vi "BinanceAPI_roundToPattern.vi"(0 "Value to round":ext, 5 "Value Pattern ( only 0 or 1 - e.g.  0,001 )":dbl) -> (4 "Rounded Value":dbl, 6 "dokladnosc zaokraglenia":i32)   [LabVIEW 2022 SP3]
doc: "Program dodatkowy\n\n\nProgram ten zaokrągla liczbę <B>Value to round</B> do tego miejsca po przecinku co podany przykład czyli <B>Value Pattern</B>"
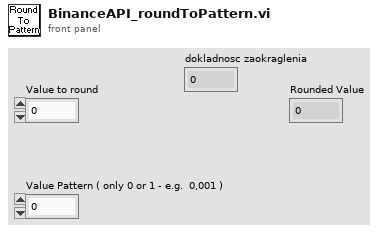
[diagram p1: front panel]
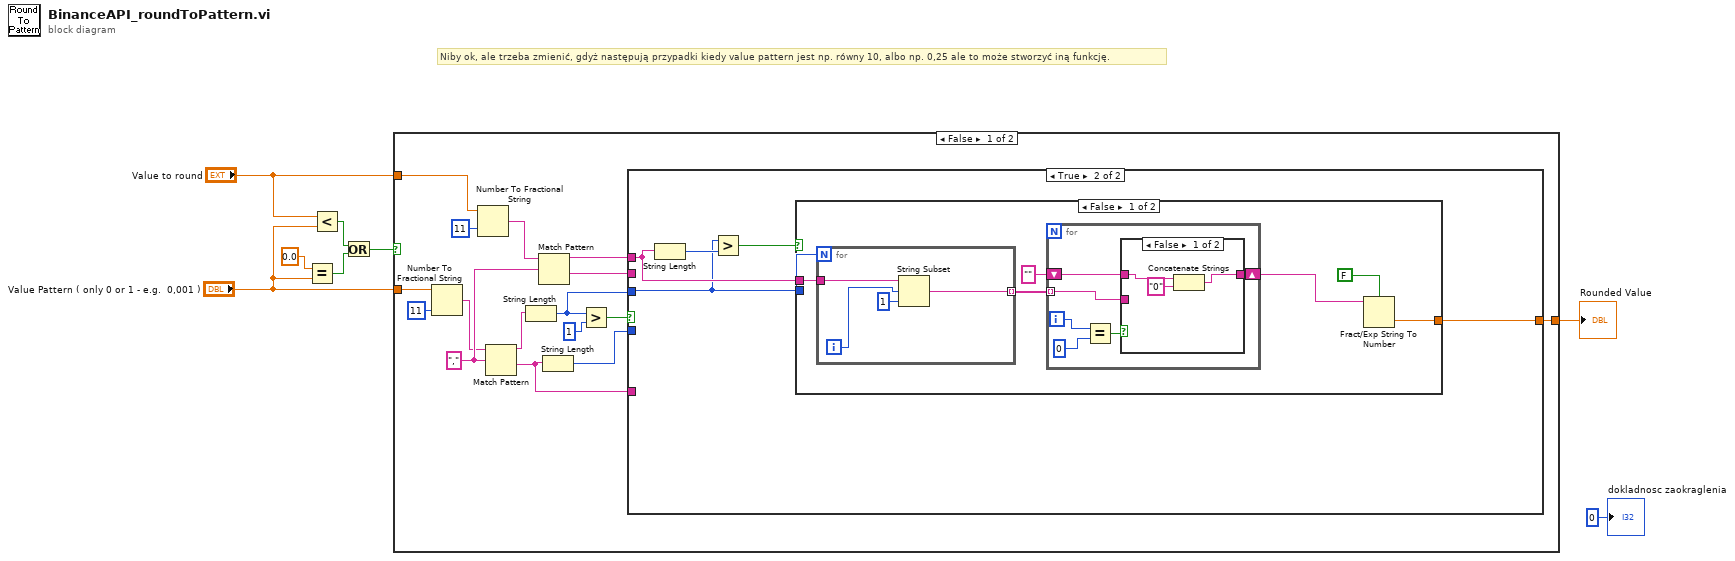
[diagram p0: block diagram]
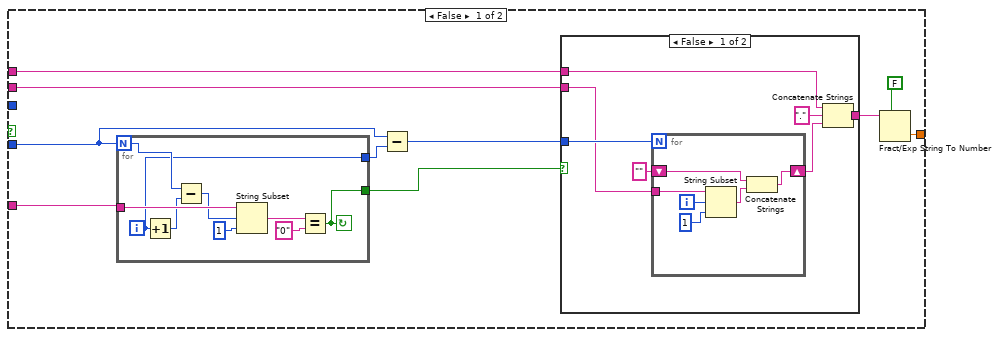
[diagram p2: hidden frame]
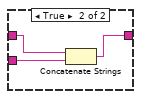
[diagram p4: hidden frame]
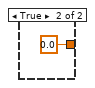
[diagram p5: hidden frame]
diagram:
  # "Niby ok, ale trzeba zmienić, gdyż następują przypadki kiedy value pattern jest np. równy 10, albo np. 0,25 ale to może stworzyć iną funkcję."
  n1 = Equal?(x=0.0 ("y"), y="Value Pattern ( only 0 or 1 - e.g.  0,001 )") -> (x = y?=w4:bool)
  n2 = Less?(x="Value to round", y="Value Pattern ( only 0 or 1 - e.g.  0,001 )") -> (x < y?=w3:bool)
  n3 = Or(x=w3, y=w4) -> (x .or. y?=w2:bool)
  n4 = case shown="False" w2 {
    tunnel: [w22 w87] -> w8
    tunnel: "Value to round" -> [w17 _]
    tunnel: "Value Pattern ( only 0 or 1 - e.g.  0,001 )" -> [w15 w87]
    frame False {
      w24 = "," ("regular expression")
      n5 = Number To Fractional String(number=w15, precision (6)=i16 11 ("width (-)")) -> (F-format string=w19:string)  [unwired: 2 in]
      n6 = Number To Fractional String(number=w17, precision (6)=i16 11 ("width (-)")) -> (F-format string=w18:string)  [unwired: 2 in]
      n7 = Match Pattern(string=w19, regular expression=w24) -> (before substring=w13:string, after substring=w20:string)  [unwired: 1 in, 2 out]
      n8 = String Length(string=w13) -> (length=w10:i32)
      n9 = Match Pattern(string=w18, regular expression=w24) -> (before substring=w14:string, after substring=w21:string)  [unwired: 1 in, 2 out]
      n10 = String Length(string=w20) -> (length=w9:i32)
      n11 = Greater?(x=w10, y=1) -> (0:w11:bool)
      n12 = case shown="True" w11 {
        tunnel: [w34 w62] -> w22
        tunnel: w21 -> [w31 _]
        tunnel: w9 -> [w30 _]
        tunnel: w20 -> [w29 _]
        tunnel: w14 -> [w26 w61]
        tunnel: w10 -> [_ w58]
        frame False {
          n13 = for {
            N: w30 -> [w52]
            tunnel: w29 -> [w57]
            tunnel: [w50] -> w28
            tunnel: [w49] -> w27
            i -> [w50]
            stop <- w49 continue-if-true
            n14 = Increment(x=w50) -> (x+1=w51:i32)
            n15 = Subtract(x=w52, y=w51) -> (x-y=w55:i32)
            n16 = String Subset(string=w57, offset (0)=w55, length (rest)=1 ("length (rest)")) -> (substring=w54:string)
            n17 = Equal?(x=w54, y="0" ("substring")) -> (x = y?=w49:bool)
          }
          n18 = Subtract(x=w30, y=w28) -> (x-y=w25:i32)
          n19 = case shown="False" w27 {
            tunnel: [w41 w48] -> w33
            tunnel: w25 -> [w39 _]
            tunnel: w31 -> [w37 _]
            tunnel: w26 -> [w36 w48]
            frame False {
              n20 = for {
                N: w39 -> [_]
                tunnel: w37 -> [w47]
                shift-right: [w42] -> w35
                shift-left: "" ("regular expression") -> [w44]
                i -> [w46]
                n21 = String Subset(string=w47, offset (0)=w46, length (rest)=1 ("length (rest)")) -> (substring=w43:string)
                n22 = Concatenate Strings(w44, w43) -> (w42:string)
              }
              n23 = Concatenate Strings(w36, "." ("regular expression"), w35) -> (w41:string)
            }
            frame True {
            }
          }
          n24 = Fract/Exp String To Number(use system decimal point (T)=FALSE, string=w33) -> (number=w34:dbl)  [unwired: 2 in, 1 out]
        }
        frame True {
          n25 = String Length(string=w61) -> (length=w60:i32)
          n26 = Greater?(x=w58, y=w60) -> (0:w59:bool)
          n27 = case shown="False" w59 {
            tunnel: [w65 0.0] -> w62
            tunnel: w61 -> [w64 _]
            tunnel: w58 -> [w63 _]
            frame False {
              n28 = for {
                N: w63 -> [_]
                tunnel: w64 -> [w84]
                tunnel: [w82] -> w69 mode=indexing
                i -> [w83]
                n29 = String Subset(string=w84, offset (0)=w83, length (rest)=1 ("length (rest)")) -> (substring=w82:string)
              }
              n30 = for {
                tunnel: w69 -> [w70] mode=indexing
                shift-right: [w71] -> w66
                shift-left: "" -> [w72]
                i -> [w75]
                n31 = Equal?(x=w75, y=0) -> (x = y?=w73:bool)
                n32 = case shown="False" w73 {
                  tunnel: w72 -> [w78 w81]
                  tunnel: [w76 w79] -> w71
                  tunnel: w70 -> [_ w80]
                  frame False {
                    n33 = Concatenate Strings(w78, "0" ("string")) -> (w76:string)
                  }
                  frame True {
                    n34 = Concatenate Strings(w81, w80) -> (w79:string)
                  }
                }
              }
              n35 = Fract/Exp String To Number(use system decimal point (T)=FALSE, string=w66) -> (number=w65:dbl)  [unwired: 2 in, 1 out]
            }
            frame True {
            }
          }
        }
      }
    }
    frame True {
    }
  }
  "Rounded Value" <- w8
  "dokladnosc zaokraglenia" <- 0 ("dokladnosc zaokraglenia")
